vi "Write Current Sense Resistivity.vi"(8 "error in (no error)":errorcluster, 10 "Array":dbl[](array[numeric]), 11 "configuration file path":path) -> (0 "error out":errorcluster, 3 "file path":path)   [LabVIEW 2023]
uses:
  <vilib>/Utility/config.llb/Write Key (Double).vi
  <vilib>/Utility/config.llb/NI_LVConfig.lvlib
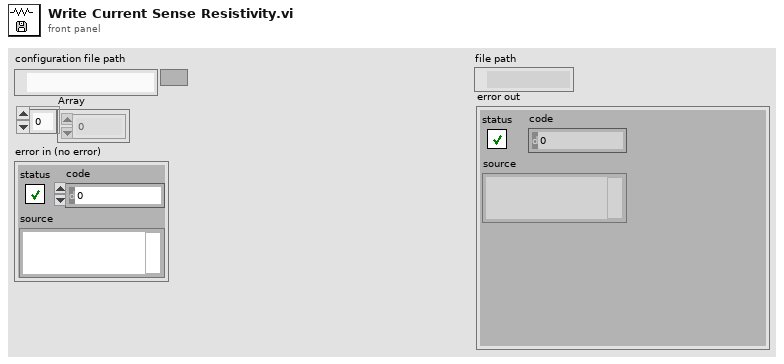
[diagram p1: front panel]
types:
  T1 = typedef "NI_LVConfig.lvlib/Config Data RefNum.ctl" = refnum<k1>
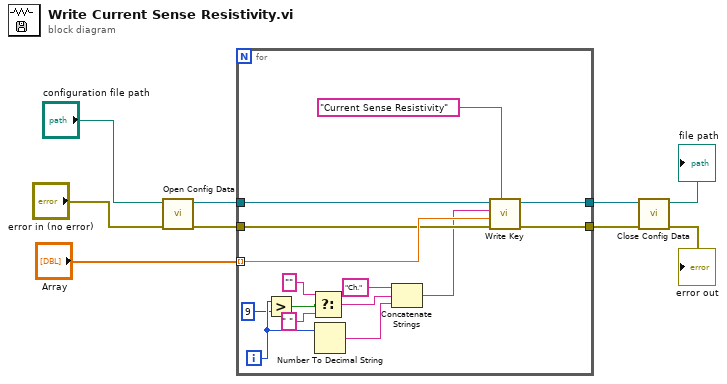
[diagram p0: block diagram]
diagram:
  n1 = call <vilib>:"Open Config Data.vi"("error in (no error)"="error in (no error)", "configuration file path"="configuration file path") -> ("error out"=w5:errorcluster, "refnum"=w4:T1)  [unwired: 7 in, 1 out]
  n2 = for {
    tunnel: [w23] -> w9
    tunnel: [w22] -> w8
    tunnel: "Array" -> [w21] mode=indexing
    tunnel: w5 -> [w19]
    tunnel: w4 -> [w18]
    i -> [w14]
    n3 = Greater?(x=w14, y=9) -> (0:w15:bool)
    n4 = Select(t="" ("string"), s=w15, f=" " ("string")) -> (s? t:f=w10:string)
    n5 = Number To Decimal String(number=w14) -> (decimal integer string=w20:string)  [unwired: 1 in]
    n6 = Concatenate Strings("Ch." ("string"), w10, w20) -> (w17:string)
    n7 = call-poly <vilib>:"Write Key.vi"("section"="Current Sense Resistivity", "error in (no error)"=w19, "value"=w21, "key"=w17, "refnum"=w18) -> ("error out"=w22:errorcluster, "refnum out"=w23:T1)  [unwired: 4 in, 1 out]
  }
  n8 = call <vilib>:"Close Config Data.vi"("error in (no error)"=w8, "refnum"=w9) -> ("error out"=→"error out":errorcluster, "file path"=→"file path":path)  [unwired: 8 in]
